vi "Calculate Center.vi"(8 "Type of Assembly Tray":i32, 9 "Syringe Coordinates":dbl[](array[numeric]), 10 "Relative Coordinates":dbl[][](array[numeric]), 11 "Fiducial Measurements":dbl[][](array[numeric])) -> (3 "XYZTheta Centers":dbl[][](array[numeric]) format="%#.9g")   [LabVIEW 2021, in "Assembly Tray.lvclass"]
uses:
  Assembly Tray.lvclass
  <vilib>/Analysis/coordinate.llb/2D Cartesian Coordinate Rotation (Scalar).vi
  <vilib>/Analysis/NI_AALPro.lvlib
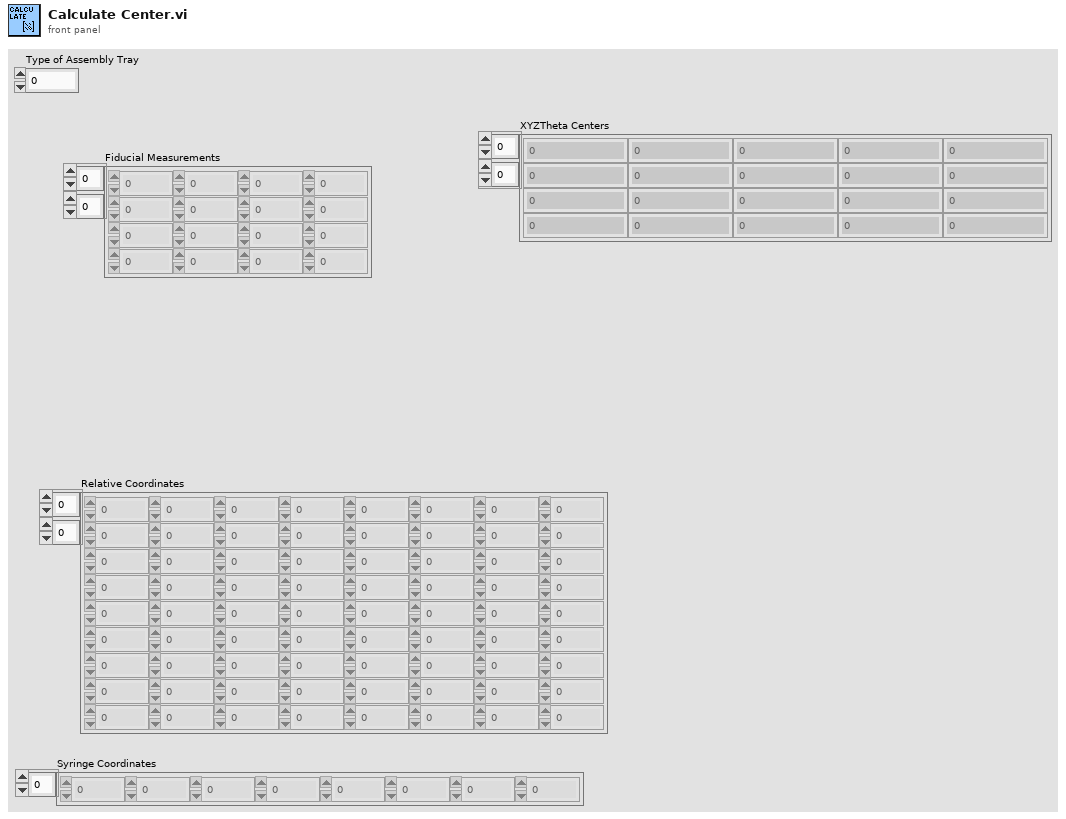
[diagram p1: front panel]
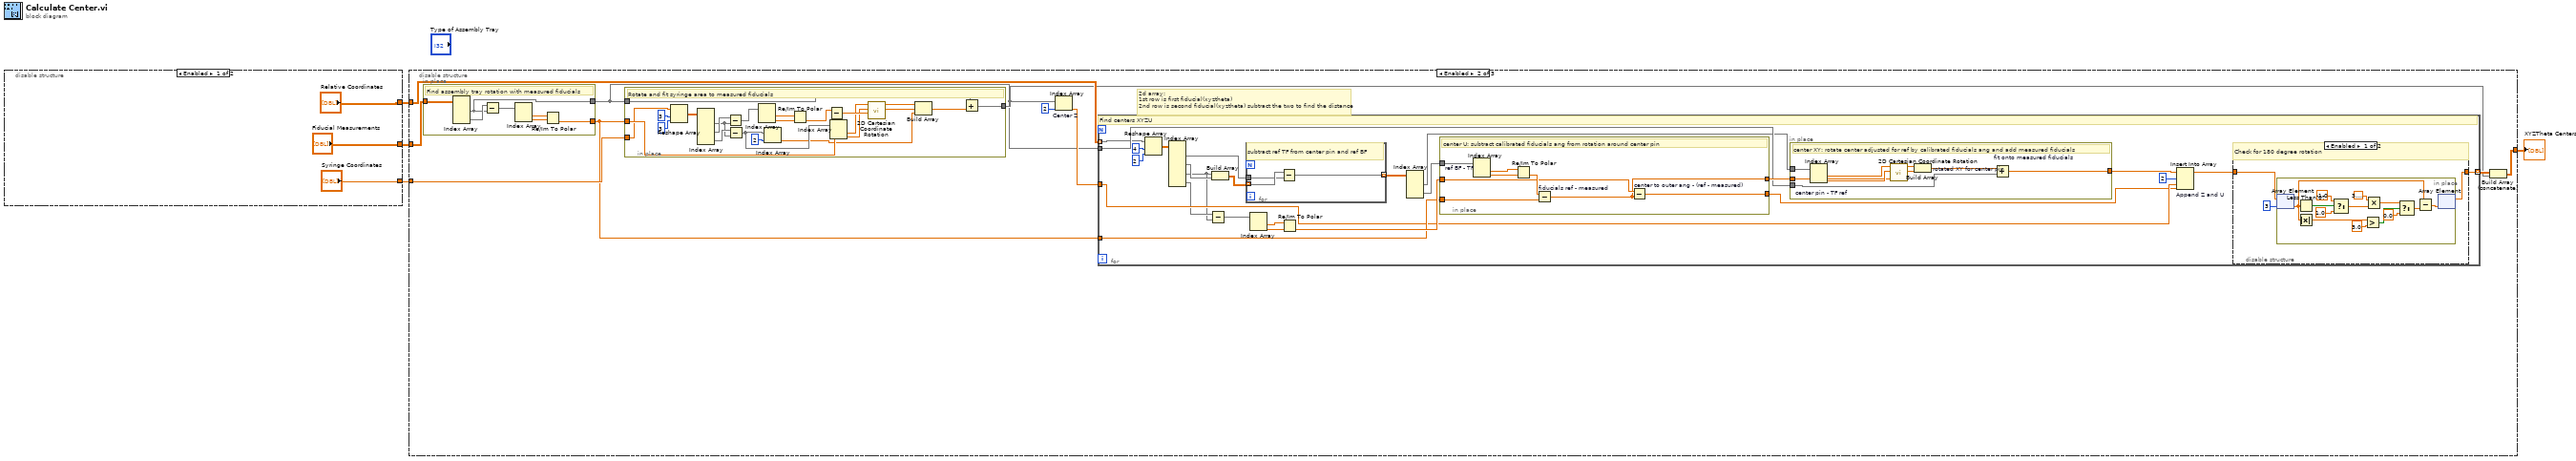
[diagram p0: block diagram]
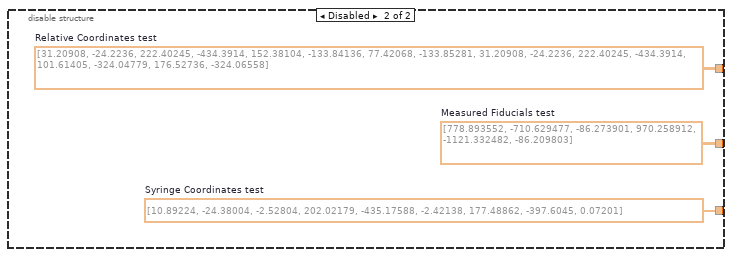
[diagram p2: hidden frame]
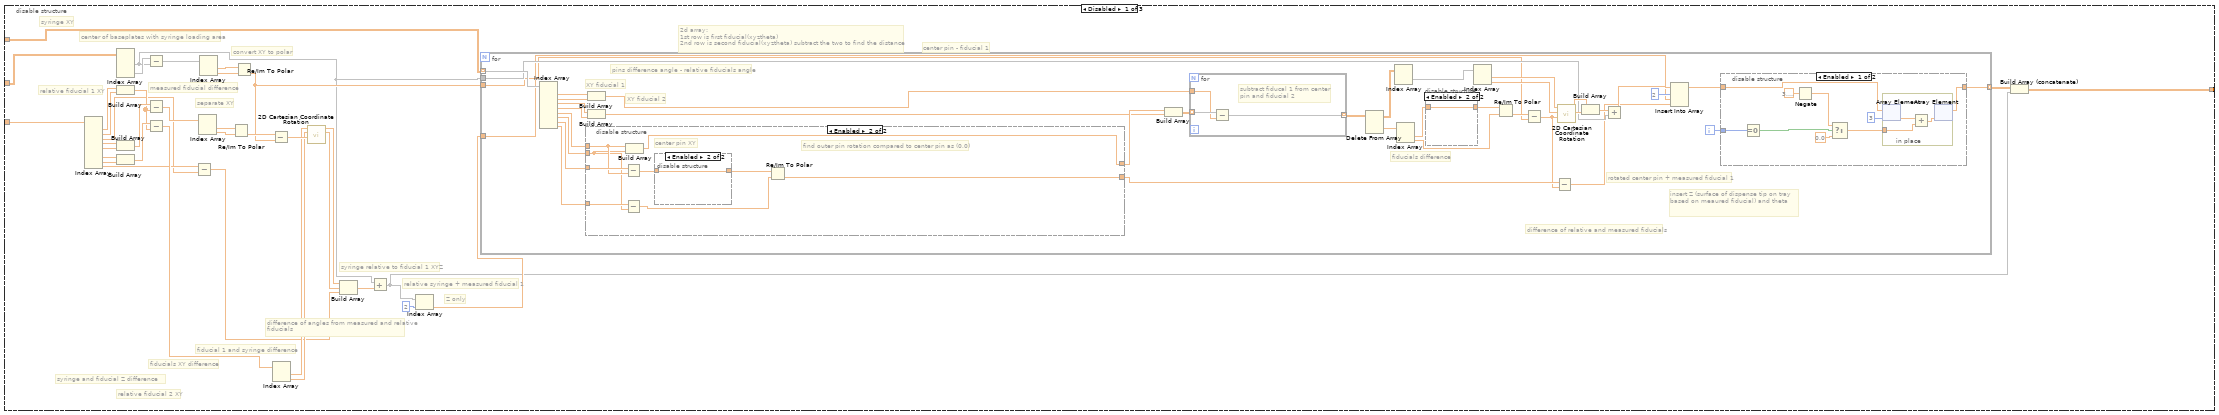
[diagram p3: hidden frame]
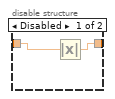
[diagram p4: hidden frame]
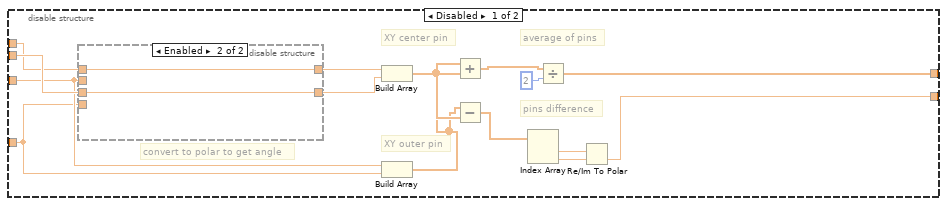
[diagram p5: hidden frame]
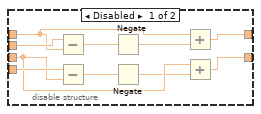
[diagram p6: hidden frame]
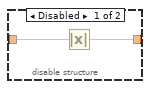
[diagram p7: hidden frame]
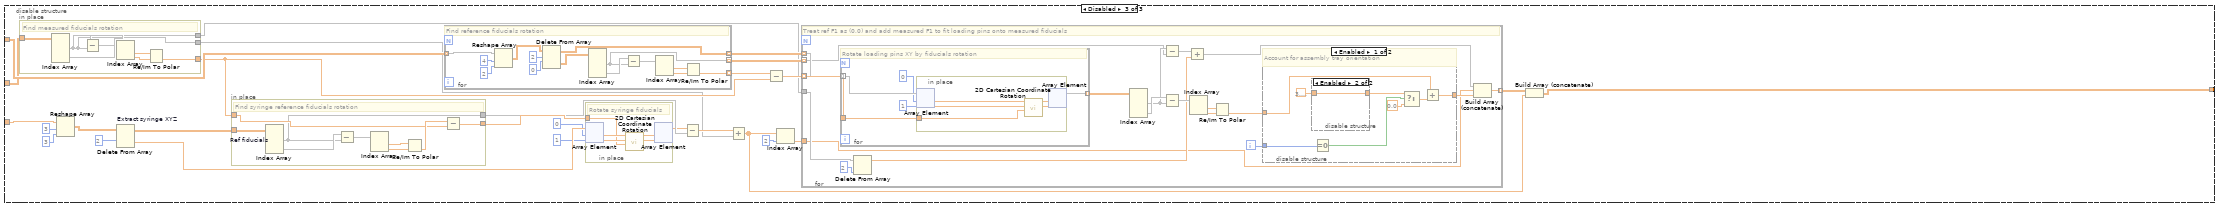
[diagram p10: hidden frame]
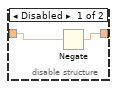
[diagram p11: hidden frame]
diagram:
  n1 = disable-structure shown="Enabled" {
    disable-tunnel: ["Syringe Coordinates" w8] -> w3
    disable-tunnel: ["Fiducial Measurements" w9] -> w2
    disable-tunnel: ["Relative Coordinates" w10] -> w1
    frame Enabled {
    }
    frame Disabled {
      w8 = dbl[] [10.89224, -24.38004, -2.52804, 202.02179, -435.17588, -2.42138, 177.48862, -397.6045, 0.07201]  # Syringe Coordinates test
      w9 = dbl[][] [[778.893552, -710.629477, -86.273901], [970.258912, -1121.332482, -86.209803]]  # Measured Fiducials test
      w10 = dbl[][] [[31.20908, -24.2236, 222.40245, -434.3914, 152.38104, -133.84136, 77.42068, -133.85281], [31.20908, -24.2236, 222.40245, -434.3914, 101.61405, -324.04779, 176.52736, -324.06558]]  # Relative Coordinates test
    }
  }
  n2 = disable-structure shown="Enabled" {
    disable-tunnel: w1 -> [w47 w152 w271]
    disable-tunnel: w2 -> [w44 w151 w270]
    disable-tunnel: w3 -> [w43 w150 w264]
    disable-tunnel: [w19 w147 w249] -> w4
    frame Disabled {
      # "center of baseplates with syringe loading area"
      # "relative fiducial 2 XY"
      # "relative fiducial 1 XY"
      # "syringe XY"
      # "center pin - fiducial 1"
      # "Z only"
      # "relative syringe + measured fiducial 1"
      # "syringe relative to fiducial 1 XYZ"
      # "difference of angles from measured and relative fiducials"
      # "separate XY"
      # "convert XY to polar"
      # "measured fiducial difference"
      # "fiducial 1 and syringe difference"
      # "syringe and fiducial Z difference"
      # "fiducials XY difference"
      # "2d array:\n1st row is first fiducial(xyztheta)\n2nd row is second fiducial(xyztheta) subtract the two to find the distance"
      n3 = Index Array(array=w43) -> (element #1=w42:dbl, element #2=w41:dbl, element #3=w23:dbl, element #4=w39:dbl, element #5=w38:dbl, element #7=w26:dbl, element #8=w25:dbl, element #9=w24:dbl)  [unwired: 9 in, 1 out]
      n4 = Index Array(array=w44) -> (element #1=w11:dbl[], element #2=w13:dbl[])  [unwired: 4 in]
      n5 = Build Array(w42, w41) -> (w30:dbl[])
      n6 = Build Array(w39, w38) -> (w40:dbl[])
      n7 = Build Array(w26, w25) -> (w31:dbl[])
      n8 = Subtract(x=w13, y=w11) -> (x-y=w18:dbl[])
      n9 = Subtract(x=w40, y=w30) -> (x-y=w37:dbl[])
      n10 = Subtract(x=w31, y=w30) -> (x-y=w29:dbl[])
      n11 = Subtract(x=w24, y=w23) -> (x-y=w15:dbl)
      n12 = Index Array(array=w37) -> (element #1=w36:dbl, element #2=w35:dbl)  [unwired: 2 in]
      n13 = Index Array(array=w18) -> (element #1=w45:dbl, element #2=w46:dbl)  [unwired: 2 in]
      n14 = Re/Im To Polar(2:w35, 3:w36) -> (0:w34:dbl)  [unwired: 1 out]
      n15 = Re/Im To Polar(2:w46, 3:w45) -> (0:w33:dbl)  [unwired: 1 out]
      n16 = Subtract(x=w34, y=w33) -> (x-y=w32:dbl)
      n17 = Index Array(array=w29) -> (element #1=w28:dbl, element #2=w27:dbl)  [unwired: 2 in]
      n18 = call-poly <vilib>:"2D Cartesian Coordinate Rotation.vi"("theta"=w32, "y"=w27, "x"=w28) -> ("y out"=w21:dbl, "x out"=w22:dbl)  [unwired: 6 in, 1 out]
      n19 = Build Array(w22, w21, w15) -> (w12:dbl[])
      n20 = Add(x=w11, y=w12) -> (x+y=w14:dbl[])
      n21 = Index Array(array=w14, index=2) -> (element=w16:dbl)
      n22 = for {
        tunnel: w47 -> [w64] mode=indexing
        tunnel: [w55] -> w20 mode=indexing
        tunnel: w11 -> [w63]
        tunnel: w33 -> [w62]
        tunnel: w16 -> [w61]
        i -> [w54]
        # "insert Z (surface of dispense tip on tray based on meaured fiducial) and theta"
        # "pins difference angle - relative fiducials angle"
        # "rotated center pin + measured fiducial 1"
        # "difference of relative and measured fiducials"
        # "fiducials difference"
        # "XY fiducial 2"
        # "XY fiducial 1"
        n23 = Index Array(array=w64) -> (element #1=w84:dbl, element #2=w83:dbl, element #3=w53:dbl, element #4=w52:dbl, element #5=w59:dbl, element #6=w60:dbl, element #7=w58:dbl, element #8=w57:dbl)  [unwired: 8 in]
        n24 = disable-structure shown="Enabled" {
          disable-tunnel: [w100 w115] -> w68
          disable-tunnel: [w94 w119] -> w66
          disable-tunnel: w60 -> [w91 w116]
          disable-tunnel: w59 -> [w90 w117]
          disable-tunnel: w58 -> [w89 w120]
          disable-tunnel: w57 -> [w88 w118]
          frame Disabled {
            # "convert to polar to get angle"
            # "pins difference"
            # "average of pins"
            # "XY outer pin"
            # "XY center pin"
            n25 = disable-structure shown="Enabled" {
              disable-tunnel: w88 -> [w112 _]
              disable-tunnel: w89 -> [w111 _]
              disable-tunnel: w91 -> [w108 w114]
              disable-tunnel: w90 -> [w105 w113]
              disable-tunnel: [w104 w114] -> w92
              disable-tunnel: [w103 w113] -> w93
              frame Disabled {
                n26 = Subtract(x=w111, y=w105) -> (x-y=w109:dbl)
                n27 = Subtract(x=w112, y=w108) -> (x-y=w110:dbl)
                n28 = Negate(x=w109) -> (-x=w106:dbl)
                n29 = Negate(x=w110) -> (-x=w107:dbl)
                n30 = Add(x=w105, y=w106) -> (x+y=w103:dbl)
                n31 = Add(x=w108, y=w107) -> (x+y=w104:dbl)
              }
              frame Enabled {
              }
            }
            n32 = Build Array(w93, w92) -> (w99:dbl[])
            n33 = Build Array(w89, w88) -> (w98:dbl[])
            n34 = Add(x=w98, y=w99) -> (x+y=w101:dbl[])
            n35 = Subtract(x=w98, y=w99) -> (x-y=w97:dbl[])
            n36 = Index Array(array=w97) -> (element #1=w96:dbl, element #2=w95:dbl)  [unwired: 2 in]
            n37 = Divide(x=w101, y=2) -> (x/y=w100:dbl[])
            n38 = Re/Im To Polar(2:w95, 3:w96) -> (0:w94:dbl)  [unwired: 1 out]
          }
          frame Enabled {
            # "find outer pin rotation compared to center pin as (0,0)"
            # "center pin XY"
            n39 = Subtract(x=w120, y=w117) -> (x-y=w122:dbl)
            n40 = Subtract(x=w118, y=w116) -> (x-y=w123:dbl)
            n41 = Build Array(w117, w116) -> (w115:dbl[])
            n42 = disable-structure shown="Enabled" {
              disable-tunnel: w122 -> [w125 w126]
              disable-tunnel: [w124 w126] -> w121
              frame Disabled {
                n43 = Absolute Value(x=w125) -> (abs(x)=w124:dbl)
              }
              frame Enabled {
              }
            }
            n44 = Re/Im To Polar(2:w123, 3:w121) -> (0:w119:dbl)  [unwired: 1 out]
          }
        }
        n45 = Build Array(w84, w83) -> (w81:dbl[])
        n46 = Build Array(w53, w52) -> (w51:dbl[])
        n47 = Build Array(w68, w51) -> (w82:dbl[][])
        n48 = for {
          tunnel: w82 -> [w142] mode=indexing
          tunnel: w81 -> [w141]
          tunnel: [w140] -> w80 mode=indexing
          # "subtract fiducal 1 from center pin and fiducial 2"
          n49 = Subtract(x=w142, y=w141) -> (x-y=w140:dbl[])
        }
        n50 = Delete From Array(array=w80) -> (deleted portion=w79:dbl[], array with subset deleted=w77:dbl[][])  [unwired: 3 in]
        n51 = Index Array(array=w77) -> (element=w76:dbl[])  [unwired: 2 in]
        n52 = Index Array(array=w79) -> (element #1=w50:dbl, element #2=w78:dbl)  [unwired: 2 in]
        n53 = disable-structure shown="Enabled" {
          disable-tunnel: w50 -> [w86 w87]
          disable-tunnel: [w85 w87] -> w49
          frame Disabled {
            n54 = Absolute Value(x=w86) -> (abs(x)=w85:dbl)
          }
          frame Enabled {
          }
        }
        n55 = Index Array(array=w76) -> (element #1=w75:dbl, element #2=w74:dbl)  [unwired: 2 in]
        n56 = Re/Im To Polar(2:w78, 3:w49) -> (0:w67:dbl)  [unwired: 1 out]
        n57 = Subtract(x=w67, y=w62) -> (x-y=w65:dbl)
        n58 = Subtract(x=w66, y=w65) -> (x-y=w48:dbl)
        n59 = call-poly <vilib>:"2D Cartesian Coordinate Rotation.vi"("theta"=w65, "y"=w74, "x"=w75) -> ("y out"=w71:dbl, "x out"=w72:dbl)  [unwired: 6 in, 1 out]
        n60 = Build Array(w72, w71) -> (w73:dbl[])
        n61 = Add(x=w73, y=w63) -> (x+y=w70:dbl[])
        n62 = Insert Into Array(array=w70, index=2, new element #1=w61, new element #2=w48) -> (w56:dbl[])
        n63 = disable-structure shown="Enabled" {
          disable-tunnel: w56 -> [w135 w139]
          disable-tunnel: [w134 w139] -> w55
          disable-tunnel: w54 -> [w132 _]
          frame Enabled {
            n64 = Equal To 0?(x=w132) -> (x = 0?=w130:bool)
            n65 = Negate(x=3.141592653589793) -> (-x=w127:dbl)
            n66 = Select(t=w127, s=w130, f=0.0) -> (s? t:f=w129:dbl)
            n67 = in-place {
              in-place-border: w129 -> [w136]
              n68 = in-place-array #1(w135, 3) -> (w138:dbl)
              n69 = Add(x=w138, y=w136) -> (x+y=w137:dbl)
              n70 = in-place-array #1(w137) -> (w134:dbl[])  [unwired: 1 out]
            }
          }
          frame Disabled {
          }
        }
      }
      n71 = Build Array (concatenate)(w20, w14) -> (w19:dbl[][])
    }
    frame Enabled {
      # "2d array:\n1st row is first fiducial(xyztheta)\n2nd row is second fiducial(xyztheta) subtract the two to find the distance"
      n72 = in-place {
        in-place-border: w151 -> [w219]
        in-place-border: [w218] -> w149
        in-place-border: [w215] -> w143
        # "Find assembly tray rotation with measured fiducials"
        n73 = Index Array(array=w219) -> (element #1=w215:dbl[], element #2=w216:dbl[])  [unwired: 4 in]
        n74 = Subtract(x=w216, y=w215) -> (x-y=w217:dbl[])
        n75 = Index Array(array=w217) -> (element #1=w220:dbl, element #2=w221:dbl)  [unwired: 2 in]
        n76 = Re/Im To Polar(2:w221, 3:w220) -> (0:w218:dbl)  [unwired: 1 out]
      }
      n77 = in-place {
        in-place-border: w150 -> [w232]
        in-place-border: w149 -> [w241]
        in-place-border: [w235] -> w144
        in-place-border: w143 -> [w233]
        # "Rotate and fit syringe area to measured fiducials"
        n78 = Reshape Array(w232, 3 ("dimension size"), 3 ("dimension size")) -> (w229:dbl[][])
        n79 = Index Array(array=w229) -> (element #1=w226:dbl[], element #2=w228:dbl[], element #3=w227:dbl[])  [unwired: 6 in]
        n80 = Subtract(x=w228, y=w226) -> (x-y=w225:dbl[])
        n81 = Subtract(x=w227, y=w226) -> (x-y=w224:dbl[])
        n82 = Index Array(array=w225) -> (element #1=w244:dbl, element #2=w243:dbl)  [unwired: 2 in]
        n83 = Index Array(array=w224, index=2) -> (element=w222:dbl)
        n84 = Re/Im To Polar(2:w243, 3:w244) -> (0:w242:dbl)  [unwired: 1 out]
        n85 = Subtract(x=w242, y=w241) -> (x-y=w240:dbl)
        n86 = Index Array(array=w224) -> (element #1=w239:dbl, element #2=w238:dbl)  [unwired: 2 in]
        n87 = call-poly <vilib>:"2D Cartesian Coordinate Rotation.vi"("theta"=w240, "y"=w238, "x"=w239) -> ("y out"=w236:dbl, "x out"=w237:dbl)  [unwired: 6 in, 1 out]
        n88 = Build Array(w237, w236, w222) -> (w234:dbl[])
        n89 = Add(x=w233, y=w234) -> (x+y=w235:dbl[])
      }
      n90 = Index Array "Center Z"(array=w144, index=2) -> (element=w145:dbl)
      n91 = for {
        tunnel: w152 -> [w166] mode=indexing
        tunnel: [w168] -> w148 mode=indexing
        tunnel: w143 -> [w172]
        tunnel: w149 -> [w171]
        tunnel: w145 -> [w170]
        # "Find centers XYZU"
        n92 = Reshape Array(w166, 4 ("dimension size"), 2 ("dimension size")) -> (w163:dbl[][])
        n93 = Index Array(array=w163) -> (element #1=w158:dbl[], element #2=w157:dbl[], element #3=w156:dbl[], element #4=w162:dbl[])  [unwired: 8 in]
        n94 = Subtract(x=w162, y=w156) -> (x-y=w161:dbl[])
        n95 = Build Array(w156, w157) -> (w177:dbl[][])
        n96 = for {
          tunnel: w177 -> [w214] mode=indexing
          tunnel: w158 -> [w213]
          tunnel: [w212] -> w155 mode=indexing
          # "subtract ref TF from center pin and ref BF"
          n97 = Subtract(x=w214, y=w213) -> (x-y=w212:dbl[])
        }
        n98 = Index Array(array=w161) -> (element #1=w160:dbl, element #2=w159:dbl)  [unwired: 2 in]
        n99 = Re/Im To Polar(2:w159, 3:w160) -> (0:w174:dbl)  [unwired: 1 out]
        n100 = Index Array(array=w155) -> (element #1=w154:dbl[], element #2=w153:dbl[])  [unwired: 4 in]
        n101 = in-place {
          in-place-border: w174 -> [w183]
          in-place-border: [w182] -> w173
          in-place-border: w171 -> [w181]
          in-place-border: [w179] -> w167
          in-place-border: w153 -> [w178]
          # "center U: subtract calibrated fiducials ang from rotation around center pin"
          n102 = Index Array "ref BF - TF"(array=w178) -> (element #1=w180:dbl, element #2=w185:dbl)  [unwired: 2 in]
          n103 = Re/Im To Polar(2:w185, 3:w180) -> (0:w184:dbl)  [unwired: 1 out]
          n104 = Subtract "fiducials ref - measured"(x=w184, y=w181) -> (x-y=w182:dbl)
          n105 = Subtract "center to outer ang - (ref - measured)"(x=w183, y=w182) -> (x-y=w179:dbl)
        }
        n106 = in-place {
          in-place-border: [w189] -> w176
          in-place-border: w173 -> [w188]
          in-place-border: w172 -> [w187]
          in-place-border: w154 -> [w186]
          # "center XY: rotate center adjusted for ref by calibrated fiducials ang and add measured fiducials"
          n107 = Index Array "center pin - TF ref"(array=w186) -> (element #1=w194:dbl, element #2=w193:dbl)  [unwired: 2 in]
          n108 = call-poly <vilib>:"2D Cartesian Coordinate Rotation.vi"("theta"=w188, "y"=w193, "x"=w194) -> ("y out"=w190:dbl, "x out"=w191:dbl)  [unwired: 6 in, 1 out]
          n109 = Build Array "rotated XY for center pin"(w191, w190) -> (w192:dbl[])
          n110 = Add "fit onto measured fiducials"(x=w192, y=w187) -> (x+y=w189:dbl[])
        }
        n111 = Insert Into Array "Append Z and U"(array=w176, index=2, new element #1=w170, new element #2=w167) -> (w169:dbl[])
        n112 = disable-structure shown="Enabled" {
          disable-tunnel: w169 -> [w196 w211]
          disable-tunnel: [w195 w211] -> w168
          frame Enabled {
            # "Check for 180 degree rotation"
            n113 = in-place {
              n114 = in-place-array #2(w196, 3) -> (w204:dbl)
              n115 = Less Than 0?(x=w204) -> (x < 0?=w210:bool)
              n116 = Absolute Value(x=w204) -> (abs(x)=w207:dbl)
              n117 = Select(t=-1.0, s=w210, f=1.0) -> (s? t:f=w199:dbl)
              n118 = Greater?(x=w207, y=3.0) -> (0:w205:bool)
              n119 = Multiply(x=3.141592653589793, y=w199) -> (x*y=w198:dbl)
              n120 = Select(t=w198, s=w205, f=0.0) -> (s? t:f=w201:dbl)
              n121 = Subtract(x=w204, y=w201) -> (x-y=w203:dbl)
              n122 = in-place-array #2(w203) -> (w195:dbl[])  [unwired: 1 out]
            }
          }
          frame Disabled {
          }
        }
      }
      n123 = Build Array (concatenate)(w148, w144) -> (w147:dbl[][])
    }
    frame Disabled {
      n124 = in-place {
        in-place-border: w270 -> [w286]
        in-place-border: [w288] -> w261
        in-place-border: [w287] -> w265
        in-place-border: [w287] -> w251
        # "Find measured fiducials rotation"
        n125 = Index Array(array=w286) -> (element #1=w287:dbl[], element #2=w292:dbl[])  [unwired: 4 in]
        n126 = Subtract(x=w292, y=w287) -> (x-y=w291:dbl[])
        n127 = Index Array(array=w291) -> (element #1=w290:dbl, element #2=w289:dbl)  [unwired: 2 in]
        n128 = Re/Im To Polar(2:w289, 3:w290) -> (0:w288:dbl)  [unwired: 1 out]
      }
      n129 = Reshape Array(w264, 3 ("dimension size"), 3 ("dimension size")) -> (w260:dbl[][])
      n130 = Delete From Array "Extract syringe XYZ"(array=w260, index (row)=2) -> (deleted portion=w257:dbl[], array with subset deleted=w258:dbl[][])  [unwired: 2 in]
      n131 = in-place {
        in-place-border: w261 -> [w280]
        in-place-border: w258 -> [w279]
        in-place-border: [w278] -> w254
        in-place-border: [w277] -> w253
        # "Find syringe reference fiducials rotation"
        n132 = Index Array "Ref fiducials"(array=w279) -> (element #1=w277:dbl[], element #2=w285:dbl[])  [unwired: 4 in]
        n133 = Subtract(x=w285, y=w277) -> (x-y=w284:dbl[])
        n134 = Index Array(array=w284) -> (element #1=w283:dbl, element #2=w282:dbl)  [unwired: 2 in]
        n135 = Re/Im To Polar(2:w282, 3:w283) -> (0:w281:dbl)  [unwired: 1 out]
        n136 = Subtract(x=w281, y=w280) -> (x-y=w278:dbl)
      }
      n137 = for {
        tunnel: w271 -> [w347] mode=indexing
        tunnel: [w340] -> w269 mode=indexing
        tunnel: [w339] -> w266 mode=indexing
        tunnel: [w335] -> w267 mode=indexing
        # "Find reference fiducials rotation"
        n138 = Reshape Array(w347, 4 ("dimension size"), 2 ("dimension size")) -> (w338:dbl[][])
        n139 = Delete From Array(array=w338, length=2, index (row)=0) -> (deleted portion=w334:dbl[][], array with subset deleted=w335:dbl[][])  [unwired: 1 in]
        n140 = Index Array(array=w334) -> (element #1=w339:dbl[], element #2=w344:dbl[])  [unwired: 4 in]
        n141 = Subtract(x=w344, y=w339) -> (x-y=w343:dbl[])
        n142 = Index Array(array=w343) -> (element #1=w342:dbl, element #2=w341:dbl)  [unwired: 2 in]
        n143 = Re/Im To Polar(2:w341, 3:w342) -> (0:w340:dbl)  [unwired: 1 out]
      }
      n144 = in-place {
        in-place-border: w254 -> [w274]
        # "Rotate syringe fiducials"
        n145 = in-place-array #3(w257, 0, 1) -> (w276:dbl, w275:dbl)
        n146 = call-poly <vilib>:"2D Cartesian Coordinate Rotation.vi"("theta"=w274, "y"=w275, "x"=w276) -> ("y out"=w272:dbl, "x out"=w273:dbl)  [unwired: 6 in, 1 out]
        n147 = in-place-array #3(w273, w272) -> (w250:dbl[])  [unwired: 2 out]
      }
      n148 = Subtract(x=w250, y=w253) -> (x-y=w252:dbl[])
      n149 = Add(x=w252, y=w251) -> (x+y=w247:dbl[])
      n150 = Subtract(x=w269, y=w261) -> (x-y=w268:dbl[])
      n151 = Index Array(array=w247, index=2) -> (element=w245:dbl)
      n152 = for {
        tunnel: w268 -> [w311] mode=indexing
        tunnel: w267 -> [w310] mode=indexing
        tunnel: [w304] -> w248 mode=indexing
        tunnel: w266 -> [w297] mode=indexing
        tunnel: w265 -> [w296]
        tunnel: w245 -> [w293]
        i -> [w303]
        # "Treat ref F1 as (0,0) and add measured F1 to fit loading pins onto measured fiducials"
        n153 = for {
          tunnel: w311 -> [w328]
          tunnel: w310 -> [w327] mode=indexing
          tunnel: [w324] -> w309 mode=indexing
          # "Rotate loading pins XY by fiducials rotation"
          n154 = in-place {
            in-place-border: w328 -> [w333]
            n155 = in-place-array #4(w327, 0, 1) -> (w332:dbl, w331:dbl)
            n156 = call-poly <vilib>:"2D Cartesian Coordinate Rotation.vi"("theta"=w333, "y"=w331, "x"=w332) -> ("y out"=w329:dbl, "x out"=w330:dbl)  [unwired: 6 in, 1 out]
            n157 = in-place-array #4(w330, w329) -> (w324:dbl[])  [unwired: 2 out]
          }
        }
        n158 = Delete From Array(array=w296, index=2) -> (array with subset deleted=w294:dbl[])  [unwired: 1 in, 1 out]
        n159 = Index Array(array=w309) -> (element #1=w298:dbl[], element #2=w308:dbl[])  [unwired: 4 in]
        n160 = Subtract(x=w298, y=w297) -> (x-y=w300:dbl[])
        n161 = Subtract(x=w308, y=w298) -> (x-y=w307:dbl[])
        n162 = Add(x=w300, y=w294) -> (x+y=w299:dbl[])
        n163 = Index Array(array=w307) -> (element #1=w306:dbl, element #2=w305:dbl)  [unwired: 2 in]
        n164 = Re/Im To Polar(2:w305, 3:w306) -> (0:w302:dbl)  [unwired: 1 out]
        n165 = disable-structure shown="Enabled" {
          disable-tunnel: w303 -> [w317 _]
          disable-tunnel: w302 -> [w316 w323]
          disable-tunnel: [w314 w323] -> w301
          frame Enabled {
            # "Account for assembly tray orientation"
            n166 = disable-structure shown="Enabled" {
              disable-tunnel: 3.141592653589793 -> [w321 w322]
              disable-tunnel: [w320 w322] -> w312
              frame Disabled {
                n167 = Negate(x=w321) -> (-x=w320:dbl)
              }
              frame Enabled {
              }
            }
            n168 = Equal To 0?(x=w317) -> (x = 0?=w319:bool)
            n169 = Select(t=w312, s=w319, f=0.0) -> (s? t:f=w315:dbl)
            n170 = Add(x=w316, y=w315) -> (x+y=w314:dbl)
          }
          frame Disabled {
          }
        }
        n171 = Build Array (concatenate)(w299, w293, w301) -> (w304:dbl[])
      }
      n172 = Build Array (concatenate)(w248, w247) -> (w249:dbl[][])
    }
  }
  "XYZTheta Centers" <- w4
